vi "CorFGV.vi"(9 "Set Size":u8, 10 "Action":T1(ring), 11 "Set Index":u8) -> (1 "Get Size":u8, 2 "Old Index":u8, 3 "Get Index":u8)   [LabVIEW 2012, in "StimulCtrls.lvlib"]
uses:
  StimulCtrls.lvlib
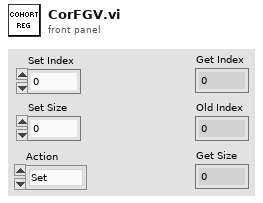
[diagram p1: front panel]
types:
  T1 = enum16{"Set", "Get", "Del", "Add", "GetSize", "SetSize"}
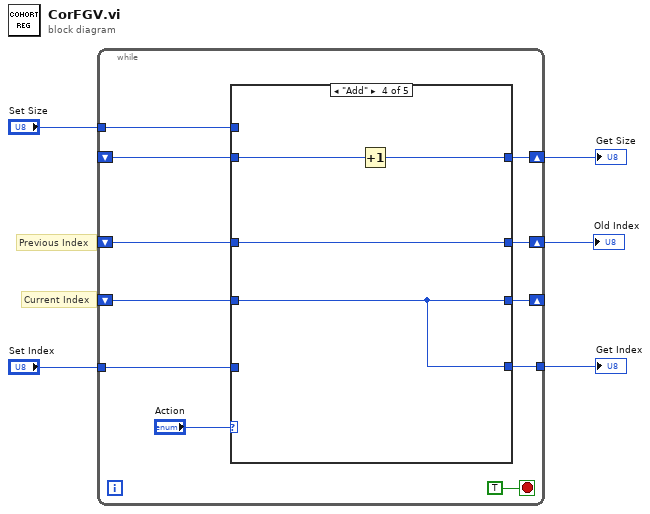
[diagram p0: block diagram]
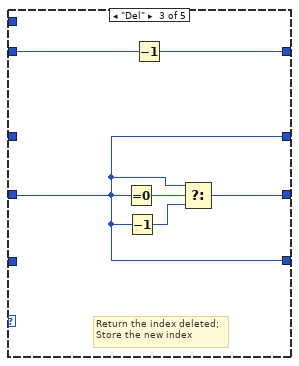
[diagram p4: hidden frame]
diagram:
  # "Current Index"
  # "Previous Index"
  n1 = while {
    tunnel: "Set Index" -> [w12]
    shift-right: [w15] -> _
    shift-left: _ -> [w14]
    tunnel: [w11] -> w4
    shift-right: [w10] -> w3
    shift-left: _ -> [w9]
    shift-right: [w8] -> w2
    shift-left: _ -> [w7]
    tunnel: "Set Size" -> [w6]
    stop <- TRUE stop-if-true
    n2 = case shown="\"Add\"" "Action" {
      tunnel: [w19 w22 w26 w30 w33] -> w15
      tunnel: w12 -> [w19 _ _ _ _]
      tunnel: w14 -> [w17 w22 w23 w30 w33]
      tunnel: [w19 w22 w23 w30 w33] -> w11
      tunnel: [w18 w21 w24 w31 w35] -> w10
      tunnel: w9 -> [w18 w21 w25 w32 _]
      tunnel: [w17 w20 w23 w29 w34] -> w8
      tunnel: w7 -> [_ w20 _ w29 w34]
      tunnel: w6 -> [_ _ _ _ w35]
      frame "Set", Default {
      }
      frame "Get" {
      }
      frame "Del" {
        # "Return the index deleted;\nStore the new index"
        n3 = Equal To 0?(x=w23) -> (x = 0?=w28:bool)
        n4 = Decrement(x=w23) -> (x-1=w27:u8)
        n5 = Decrement(x=w25) -> (x-1=w24:u8)
        n6 = Select(t=w23, s=w28, f=w27) -> (s? t:f=w26:u8)
      }
      frame "Add" {
        n7 = Increment(x=w32) -> (x+1=w31:u8)
      }
      frame "SetSize" {
      }
    }
  }
  "Get Index" <- w4
  "Get Size" <- w3
  "Old Index" <- w2
